vi "Autonomous Independent.vi"() -> ()   [LabVIEW 2015]
doc: "This VI is called when autonomous begins, and will automatically be terminated when autonomous ends. You can carry out timed or sensor driven robot movement independently without needing to return to the caller."
uses:
  Robot Global Data.vi
  <vilib>/Rock Robotics/Network Tables/NT Read Number.vi
  <vilib>/Rock Robotics/Network Tables/NT Read Boolean.vi
panel:
  out "Right Inches":dbl
  out "left inches":dbl
  out "Gyro Angle":dbl
  # "Be sure to right-click and choose Data Operations>>Make Current Value default if you want to save the array values with the VI"
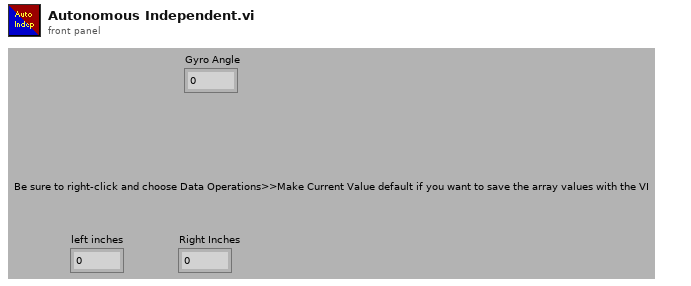
[diagram p1: front panel]
types:
  T1 = typedef "WPI_MotorControlDeviceRef.ctl" = cluster{"DeviceStatus":errorcluster, "Type":T2, "PWM":cluster{"PWM Channel":T3, "DeadBand":T4}, "CAN":cluster{"Device Number":u8, "Control Mode":T5, "Semaphore":T6, "Max Vout":dbl, "TalonSRX Control Mode":T7}, "Invert":bool}
  T2 = typedef "WPI_MotorControlType.ctl" = enum16{"PWM", "CAN", "CANTalonSRX"}
  T3 = typedef "FPGA_DIOPWMChannel.ctl" = enum8{"PWM 0", "PWM 1", "PWM 2", "PWM 3", "PWM 4", "PWM 5", "PWM 6", "PWM 7", "PWM 8", "PWM 9", "PWM MXP 0", "PWM MXP 1", "PWM MXP 2", "PWM MXP 3", "PWM MXP 4", "PWM MXP 5", "PWM MXP 6", "PWM MXP 7", "PWM MXP 8", "PWM MXP 9", "Invalid"}
  T4 = typedef "WPI_PWMDeadband.ctl" = cluster{"Name":string, "maxPositivePwm":i32, "minPositivePwm":i32, "centerPwm":i32, "maxNegativePwm":i32, "minNegativePwm":i32, "angularRange":u16}
  T5 = typedef "WPI_CANJaguar_ControlMode.ctl" = enum8{"Percent VBus", "Current", "Speed", "Position", "Voltage"}
  T6 = typedef "Semaphore RefNum" = refnum<k1>
  T7 = typedef "WPI_CANTalonSRX_APIControlMode.ctl" = enum8{"Percent VBus", "Speed", "Position", "Slave", "Unchanged / Invalid", "Voltage Compensation", "Current", "Motion Profile"}
  T8 = typedef "WPI_GyroDevRef.ctl" = cluster{"DevStatus":errorcluster, "Analog Channel":T9, "Offset":dbl, "Gain (VoltsPerDegree/Second)":dbl, "Gyro Type":enum16{"Analog", "XRS450"}, "Handle":i32, "SPI Bus":T10, "Device Found":bool, "Sample Rate":dbl, "Calibrate On Open":bool}
  T9 = typedef "FPGA_AIChannel.ctl" = enum8{"AI 0", "AI 1", "AI 2", "AI 3", "AI MXP 0", "AI MXP 1", "AI MXP 2", "AI MXP 3", "Invalid"}
  T10 = typedef "spi_bus.ctl" = enum16{"SPI On-Board, CS0", "SPI On-Board, CS1", "SPI On-Board, CS2", "SPI On-Board, CS3", "SPI MXP", "Invalid"}
  T11 = typedef "WPI_CANTalonSRX_GlobalStatus.ctl" = cluster{"Applied Throttle":dbl, "Module Enabled":bool, "CAN Error":errorcluster, "Closed Loop Error":dbl, "Forward Limit Switch Closed":bool, "Reverse Limit Switch Closed":bool, "Sensor Position":dbl, "Sensor Velocity":dbl, "Current":dbl, "Sticky Fault - Over Temp":bool, "Sticky Fault - Under Voltage":bool, "Sticky Fault - Forward Limit":bool, "Sticky Fault - Reverse Limit":bool, "Sticky Fault - Forward Soft Limit":bool, "Sticky Fault - Reverse Soft Limit":bool, "Brake is Enabled":bool, "Encoder Position":dbl, "Encoder Velocity":dbl, "Encoder Index Count":dbl, "Encoder A Pin State":bool, "Encoder B Pin State":bool, "Encoder Index Pin State":bool, "Analog In":dbl, "Analog In Velocity":dbl, "Temperature (C)":dbl, "Battery Voltage":dbl, "Control 5 Is Supported":bool, "Current Profile Slot Select":dbl, "Pos Div 8":bool, "Vel Div 4":bool, "Pulse Width Position":i32, "Pulse Width Velocity":i32, "Pulse Width Rise To Rise (us)":i32, "Pulse Width Rise To Fall (us)":i32, "Mot Prof Active Is Under Run":bool, "Mot Prof Active Has Under Run":bool, "Mot Prof Active Is Last":bool, "Mot Prof Active Velocity Only":bool, "Mot Prof Active Is Valid":bool, "Mot Prof Buffer Is Full":bool, "Mot Prof Active Profile Slot Select":i32, "Mot Prof NextID":i32, "Mot Prof Count":i32, "Mot Prof Active Velocity":dbl, "Mot Prof Active Position":dbl, "Mot Prof Output Enable":i32}
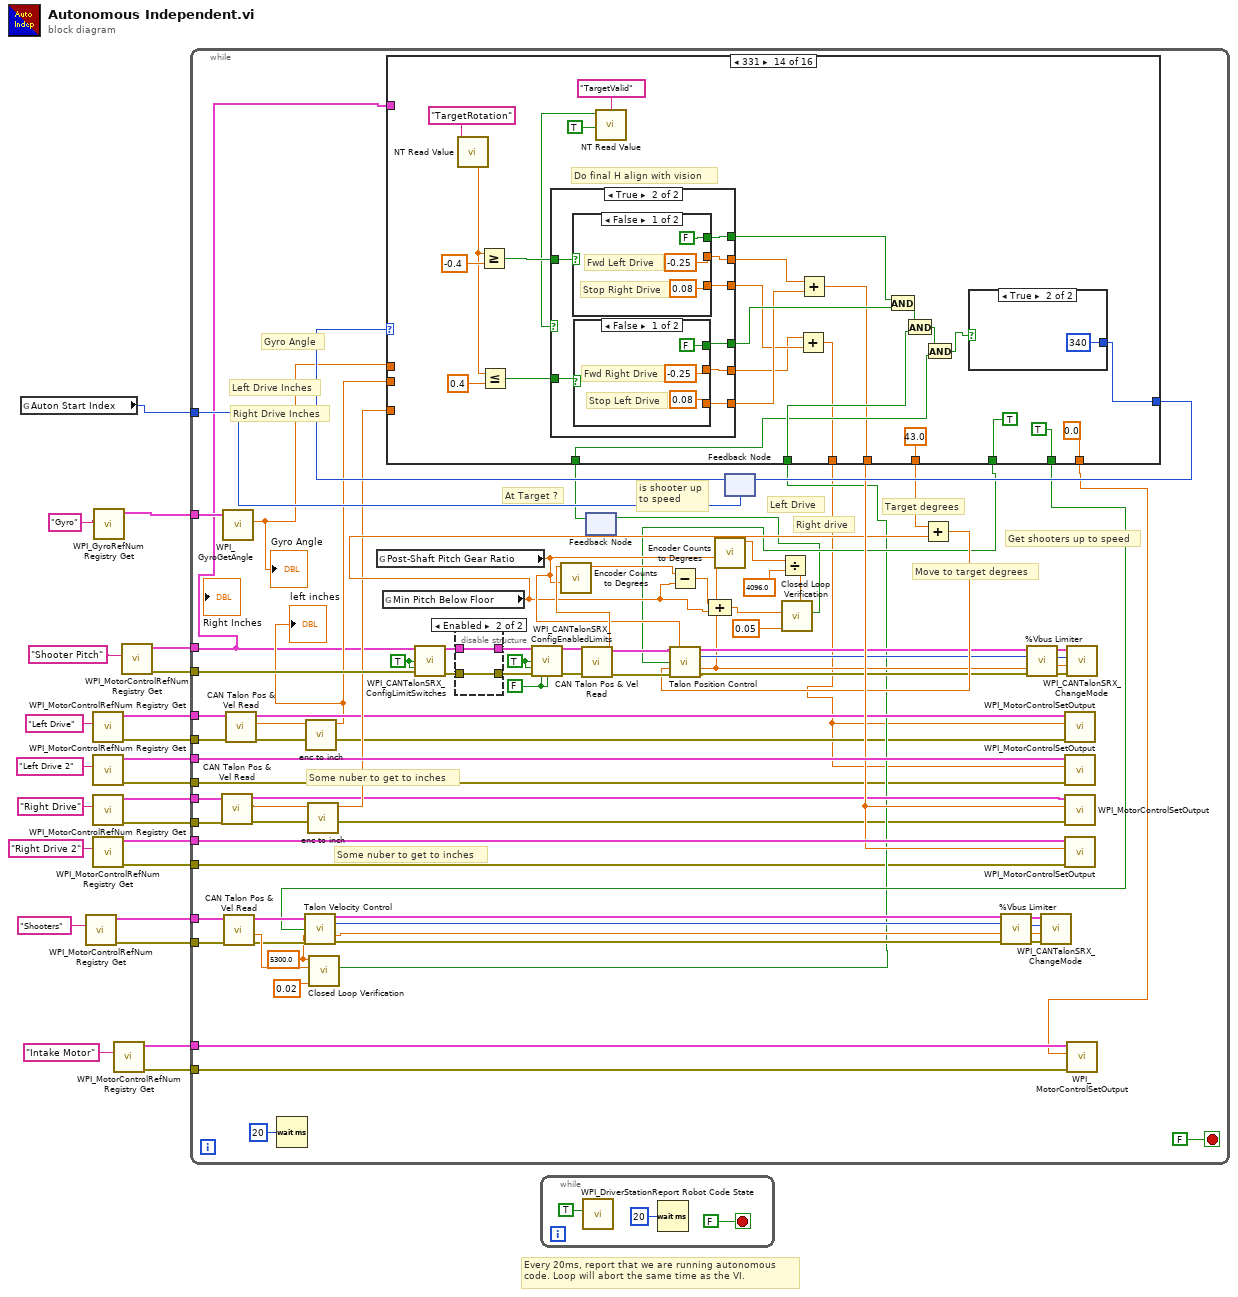
[diagram p0: block diagram]
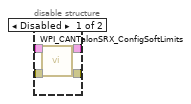
[diagram p2: hidden frame]
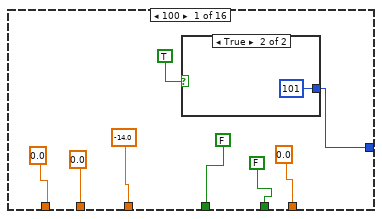
[diagram p3: hidden frame]
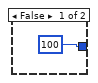
[diagram p4: hidden frame]
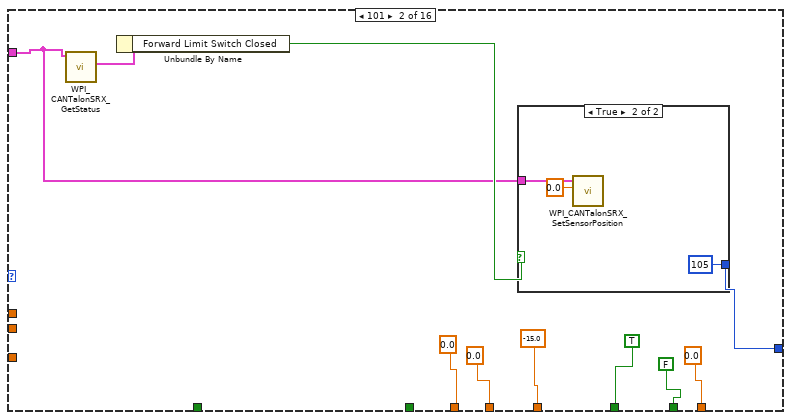
[diagram p5: hidden frame]
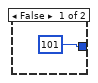
[diagram p6: hidden frame]
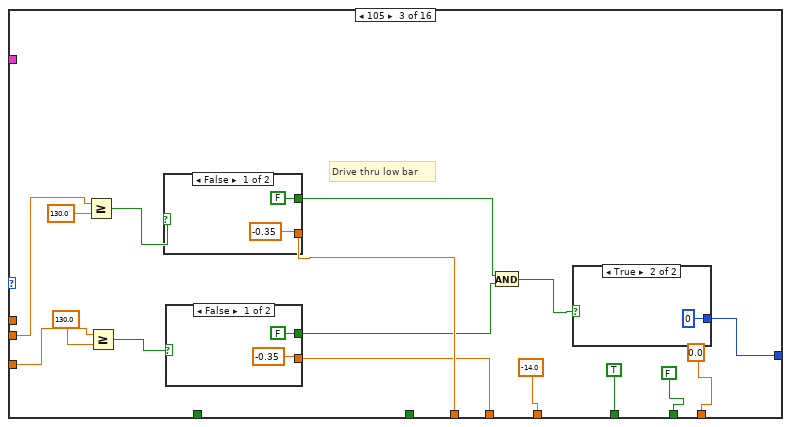
[diagram p7: hidden frame]
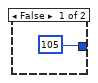
[diagram p8: hidden frame]
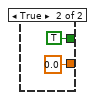
[diagram p9: hidden frame]
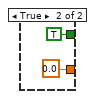
[diagram p10: hidden frame]
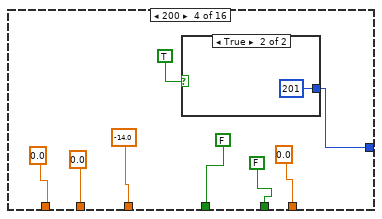
[diagram p11: hidden frame]
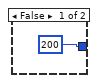
[diagram p12: hidden frame]
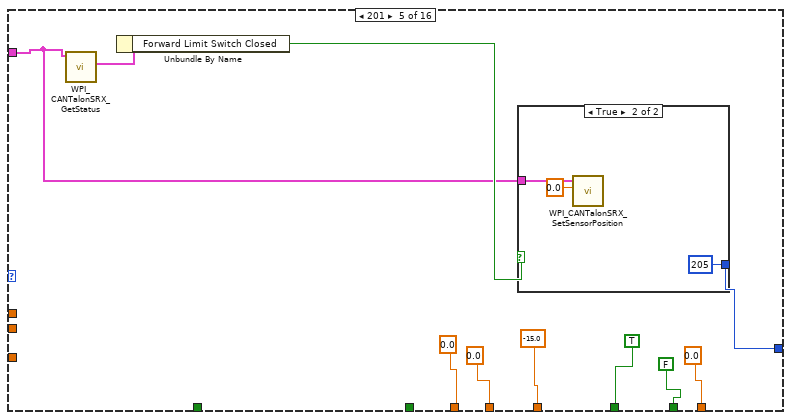
[diagram p13: hidden frame]
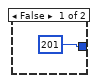
[diagram p14: hidden frame]
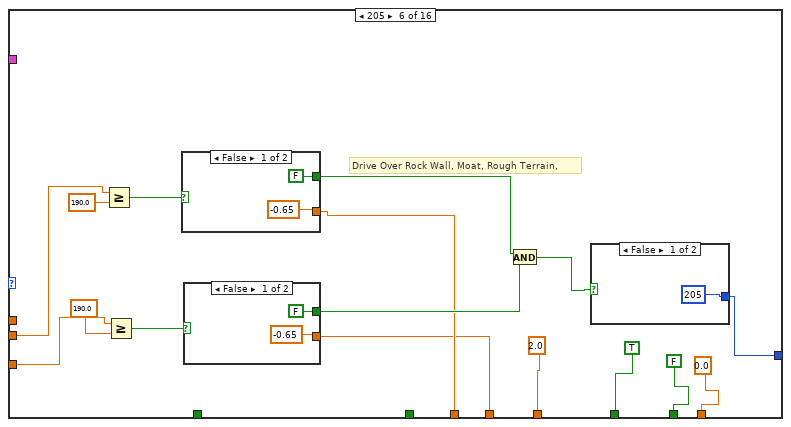
[diagram p15: hidden frame]
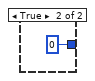
[diagram p16: hidden frame]
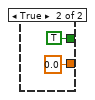
[diagram p17: hidden frame]
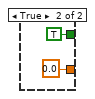
[diagram p18: hidden frame]
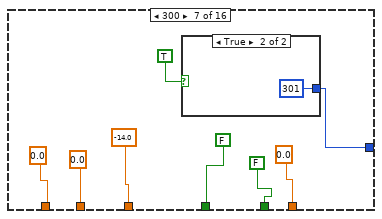
[diagram p19: hidden frame]
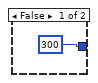
[diagram p20: hidden frame]
diagram:
  # "Every 20ms, report that we are running autonomous\ncode. Loop will abort the same time as the VI."
  n1 = global read "Robot Global Data.vi" "Auton Start Index"() -> (w1:i32)
  n2 = call <vilib>:"WPI_MotorControlRefNum Registry Get.vi"("refnum name"="Shooters") -> ("error out"=w7:errorcluster, "MotorControlDevRef"=w8:T1)  [unwired: 9 in]
  n3 = call <vilib>:"WPI_MotorControlRefNum Registry Get.vi"("refnum name"="Left Drive") -> ("error out"=w12:errorcluster, "MotorControlDevRef"=w13:T1)  [unwired: 9 in]
  n4 = call <vilib>:"WPI_MotorControlRefNum Registry Get.vi"("refnum name"="Left Drive 2") -> ("error out"=w2:errorcluster, "MotorControlDevRef"=w20:T1)  [unwired: 9 in]
  n5 = call <vilib>:"WPI_MotorControlRefNum Registry Get.vi"("refnum name"="Right Drive") -> ("error out"=w10:errorcluster, "MotorControlDevRef"=w11:T1)  [unwired: 9 in]
  n6 = call <vilib>:"WPI_MotorControlRefNum Registry Get.vi"("refnum name"="Right Drive 2") -> ("error out"=w3:errorcluster, "MotorControlDevRef"=w19:T1)  [unwired: 9 in]
  n7 = call <vilib>:"WPI_GyroRefNum Registry Get.vi"("refnum name"="Gyro") -> ("GyroDevRef"=w15:T8)  [unwired: 9 in, 1 out]
  n8 = call <vilib>:"WPI_MotorControlRefNum Registry Get.vi"("refnum name"="Intake Motor") -> ("error out"=w4:errorcluster, "MotorControlDevRef"=w5:T1)  [unwired: 9 in]
  n9 = call <vilib>:"WPI_MotorControlRefNum Registry Get.vi"("refnum name"="Shooter Pitch") -> ("error out"=w16:errorcluster, "MotorControlDevRef"=w17:T1)  [unwired: 9 in]
  n10 = while {
    tunnel: w1 -> [w101]
    tunnel: w15 -> [w100]
    tunnel: w13 -> [w58]
    tunnel: w20 -> [w98]
    tunnel: w11 -> [w55]
    tunnel: w19 -> [w97]
    tunnel: w17 -> [w26]
    tunnel: w16 -> [w88]
    tunnel: w12 -> [w59]
    tunnel: w10 -> [w53]
    tunnel: w8 -> [w50]
    tunnel: w7 -> [w49]
    tunnel: w5 -> [w33]
    tunnel: w4 -> [w32]
    tunnel: w3 -> [w31]
    tunnel: w2 -> [w29]
    stop <- FALSE stop-if-true
    w44 = 5300.0 ("Target")
    w89 = FALSE ("Forward Soft Limit Enable")
    w90 = TRUE ("Forward Limit Switch Enable")
    w95 = TRUE ("Forward Limit Switch Normally Open")
    # "is shooter up\nto speed"
    # "Get shooters up to speed"
    # "Right Drive Inches"
    # "Left Drive Inches"
    # "Gyro Angle"
    # "Some nuber to get to inches"
    # "Some nuber to get to inches"
    # "At Target ?"
    # "Move to target degrees"
    # "Target degrees"
    # "Right drive"
    # "Left Drive"
    n11 = call "CAN Talon Pos & Vel Read.vi"("error in (no error)"=w53, "CAN Talon SRX Ref"=w55) -> ("error out"=w30:errorcluster, "Sensor Position"=w52:dbl, "CAN Talon SRX Ref"=w54:T1)  [unwired: 5 in, 2 out]
    n12 = call <vilib>:"WPI_GyroGetAngle.vi"("GyroDevRef"=w100) -> ("Angle"=w99:dbl)  [unwired: 6 in, 4 out]
    "Gyro Angle" <- w99
    n13 = call "CAN Talon Pos & Vel Read.vi"("error in (no error)"=w49, "CAN Talon SRX Ref"=w50) -> ("error out"=w46:errorcluster, "Sensor Velocity"=w47:dbl, "CAN Talon SRX Ref"=w45:T1)  [unwired: 5 in, 2 out]
    n14 = call "CAN Talon Pos & Vel Read.vi"("error in (no error)"=w59, "CAN Talon SRX Ref"=w58) -> ("error out"=w28:errorcluster, "Sensor Position"=w57:dbl, "CAN Talon SRX Ref"=w56:T1)  [unwired: 5 in, 2 out]
    n15 = Wait (ms)(milliseconds to wait=u32 20) -> ()  [unwired: 1 out]
    n16 = call "enc to inch.vi"("Sensor position"=w57) -> ("Inches"=w51:dbl)  [unwired: 10 in]
    "left inches" <- w51
    n17 = call "enc to inch.vi"("Sensor position"=w52) -> ("Inches"=w60:dbl)  [unwired: 10 in]
    n18 = call "Closed Loop Verification.vi"("Allowable Error Factor"=0.02, "Actual"=w47, "Target"=w44) -> ("At Target w/in Allowable Error?"=w34:bool)  [unwired: 8 in]
    n19 = global read "Robot Global Data.vi" "Post-Shaft Pitch Gear Ratio"() -> (w78:dbl)
    n20 = global read "Robot Global Data.vi" "Min Pitch Below Floor"() -> (w75:dbl)
    n21 = call <vilib>:"WPI_CANTalonSRX_ConfigLimitSwitches.vi"("CAN Talon SRX Ref"=w26, "Forward Limit Switch Normally Open"=w95, "Reverse Limit Switch Normally Open"=w95, "error in (no error)"=w88) -> ("CAN Talon SRX Ref"=w94:T1, "error out"=w93:errorcluster)  [unwired: 10 in]
    n22 = disable-structure shown="Enabled" {
      disable-tunnel: w94 -> [w109 w111]
      disable-tunnel: w93 -> [w108 w110]
      disable-tunnel: [w107 w111] -> w92
      disable-tunnel: [w106 w110] -> w91
      frame Disabled {
        n23 = call <vilib>:"WPI_CANTalonSRX_ConfigSoftLimits.vi"("CAN Talon SRX Ref"=w109, "error in (no error)"=w108) -> ("CAN Talon SRX Ref"=w107:T1, "error out"=w106:errorcluster)  [unwired: 12 in]
      }
      frame Enabled {
      }
    }
    n24 = call <vilib>:"WPI_CANTalonSRX_ConfigEnabledLimits.vi"("CAN Talon SRX Ref"=w92, "Forward Limit Switch Enable"=w90, "Reverse Limit Switch Enable"=w90, "error in (no error)"=w91, "Forward Soft Limit Enable"=w89, "Reverse Soft Limit Enable"=w89) -> ("CAN Talon SRX Ref"=w87:T1, "error out"=w86:errorcluster)  [unwired: 8 in]
    n25 = call "CAN Talon Pos & Vel Read.vi"("error in (no error)"=w86, "CAN Talon SRX Ref"=w87) -> ("error out"=w82:errorcluster, "Sensor Position"=w85:dbl, "CAN Talon SRX Ref"=w83:T1)  [unwired: 5 in, 2 out]
    n26 = call "Encoder Counts to Degrees.vi"("Post-Shaft Gear Ratio"=w78, "Encoder Rotations"=w85) -> ("Degrees"=w84:dbl)  [unwired: 9 in]
    n27 = feedback #1() -> (w69:bool)  [unwired: 1 in]
    n28 = Subtract(x=w84, y=w75) -> (x-y=w81:dbl)
    n29 = Compound Arithmetic op=ADD(w81, w75) -> (w80:dbl)
    n30 = feedback #2(w101) -> (w102:i64)
    n31 = case shown="331" w102 {
      tunnel: [w117 w129 w139 w167 w179 w188 w217 w229 w238 w264 w291 w317 w345 w392 w438 i64 0 ("milliseconds to wait")] -> w103
      tunnel: w99 -> [_ _ _ _ _ _ _ _ _ _ _ _ _ _ _ _]
      tunnel: [0.0 ("Angle") 0.0 ("Angle") w146 0.0 ("Angle") 0.0 ("Angle") w192 0.0 ("Angle") 0.0 ("Angle") w242 w268 w295 w321 w349 w369 w442 0.0 ("Angle")] -> w25
      tunnel: [0.0 ("Angle") 0.0 ("Angle") w145 0.0 ("Angle") 0.0 ("Angle") w191 0.0 ("Angle") 0.0 ("Angle") w241 w267 w294 w320 w348 w368 w441 0.0 ("Angle")] -> w96
      tunnel: [-14.0 ("Angle") -15.0 ("Angle") -14.0 ("Angle") -14.0 ("Angle") -15.0 ("Angle") 2.0 ("Angle") -14.0 ("Angle") -15.0 ("Angle") -14.0 ("Angle") 43.0 ("Angle") 43.0 ("Angle") 43.0 ("Angle") 43.0 ("Angle") 43.0 ("Angle") 43.0 ("Angle") -15.8 ("Angle")] -> w76
      tunnel: [FALSE ("Forward Soft Limit Enable") TRUE ("Forward Soft Limit Enable") TRUE ("Forward Soft Limit Enable") FALSE ("Forward Soft Limit Enable") TRUE ("Forward Soft Limit Enable") TRUE ("Forward Soft Limit Enable") FALSE ("Forward Soft Limit Enable") TRUE ("Forward Soft Limit Enable") TRUE ("Forward Soft Limit Enable") TRUE ("Forward Soft Limit Enable") TRUE ("Forward Soft Limit Enable") TRUE ("Forward Soft Limit Enable") TRUE ("Forward Soft Limit Enable") TRUE ("Forward Soft Limit Enable") TRUE ("Forward Soft Limit Enable") FALSE ("Forward Soft Limit Enable")] -> w74
      tunnel: w69 -> [_ _ _ _ _ _ _ _ _ _ _ w316 w341 w385 w431 _]
      tunnel: w51 -> [_ _ w147 _ _ w193 _ _ w243 w269 w296 w322 w350 _ w443 _]
      tunnel: w60 -> [_ _ w148 _ _ w194 _ _ w244 w270 w297 w323 w351 _ w444 _]
      tunnel: [FALSE FALSE FALSE FALSE FALSE FALSE FALSE FALSE FALSE FALSE FALSE ("Forward Soft Limit Enable") FALSE ("Forward Soft Limit Enable") TRUE ("Forward Soft Limit Enable") TRUE ("Forward Soft Limit Enable") TRUE ("Forward Soft Limit Enable") FALSE ("Forward Soft Limit Enable")] -> w43
      tunnel: w34 -> [_ _ _ _ _ _ _ _ _ _ _ _ _ w390 w436 _]
      tunnel: [0.0 ("Angle") 0.0 ("Angle") 0.0 ("Angle") 0.0 ("Angle") 0.0 ("Angle") 0.0 ("Angle") 0.0 ("Angle") 0.0 ("Angle") 0.0 ("Angle") 0.0 ("Angle") 0.0 ("Angle") 0.0 ("Angle") 0.0 ("Angle") 0.0 ("Angle") 1.0 ("Angle") 0.0 ("Angle")] -> w27
      tunnel: w26 -> [_ w122 _ _ w172 _ _ w222 _ _ _ _ _ _ _ _]
      frame 100 {
        n32 = case shown="True" TRUE {
          tunnel: [i64 100 ("milliseconds to wait") i64 101 ("milliseconds to wait")] -> w117
          frame False {
          }
          frame True {
          }
        }
      }
      frame 101 {
        n33 = call <vilib>:"WPI_CANTalonSRX_GetStatus.vi"("CAN Talon SRX Ref"=w122) -> ("Talon SRX Status"=w124:T11)  [unwired: 8 in, 2 out]
        n34 = Unbundle By Name(w124) -> ("Forward Limit Switch Closed"=w123:bool)
        n35 = case shown="True" w123 {
          tunnel: [i64 101 ("milliseconds to wait") i64 105 ("milliseconds to wait")] -> w129
          tunnel: w122 -> [_ w134]
          frame False {
          }
          frame True {
            n36 = call <vilib>:"WPI_CANTalonSRX_SetSensorPosition.vi"("New Sensor Position"=0.0, "CAN Talon SRX Ref"=w134) -> ()  [unwired: 8 in, 2 out]
          }
        }
      }
      frame 105 {
        # "Drive thru low bar"
        n37 = Greater Or Equal?(x=w147, y=130.0) -> (x >= y?=w151:bool)
        n38 = Greater Or Equal?(x=w148, y=130.0) -> (x >= y?=w150:bool)
        n39 = case shown="False" w151 {
          tunnel: [-0.35 ("y") 0.0 ("y")] -> w146
          tunnel: [FALSE TRUE] -> w142
          frame False {
          }
          frame True {
          }
        }
        n40 = case shown="False" w150 {
          tunnel: [-0.35 ("y") 0.0 ("y")] -> w145
          tunnel: [FALSE TRUE] -> w141
          frame False {
          }
          frame True {
          }
        }
        n41 = And(x=w142, y=w141) -> (x .and. y?=w140:bool)
        n42 = case shown="True" w140 {
          tunnel: [i64 105 ("milliseconds to wait") i64 0 ("milliseconds to wait")] -> w139
          frame False {
          }
          frame True {
          }
        }
      }
      frame 200 {
        n43 = case shown="True" TRUE {
          tunnel: [i64 200 ("milliseconds to wait") i64 201 ("milliseconds to wait")] -> w167
          frame False {
          }
          frame True {
          }
        }
      }
      frame 201 {
        n44 = call <vilib>:"WPI_CANTalonSRX_GetStatus.vi"("CAN Talon SRX Ref"=w172) -> ("Talon SRX Status"=w174:T11)  [unwired: 8 in, 2 out]
        n45 = Unbundle By Name(w174) -> ("Forward Limit Switch Closed"=w173:bool)
        n46 = case shown="True" w173 {
          tunnel: [i64 201 ("milliseconds to wait") i64 205 ("milliseconds to wait")] -> w179
          tunnel: w172 -> [_ w184]
          frame False {
          }
          frame True {
            n47 = call <vilib>:"WPI_CANTalonSRX_SetSensorPosition.vi"("New Sensor Position"=0.0, "CAN Talon SRX Ref"=w184) -> ()  [unwired: 8 in, 2 out]
          }
        }
      }
      frame 205 {
        # "Drive Over Rock Wall, Moat, Rough Terrain,"
        n48 = Greater Or Equal?(x=w193, y=190.0) -> (x >= y?=w200:bool)
        n49 = Greater Or Equal?(x=w194, y=190.0) -> (x >= y?=w199:bool)
        n50 = case shown="False" w200 {
          tunnel: [-0.65 ("y") 0.0 ("y")] -> w192
          tunnel: [FALSE TRUE] -> w197
          frame False {
          }
          frame True {
          }
        }
        n51 = case shown="False" w199 {
          tunnel: [-0.65 ("y") 0.0 ("y")] -> w191
          tunnel: [FALSE TRUE] -> w196
          frame False {
          }
          frame True {
          }
        }
        n52 = And(x=w197, y=w196) -> (x .and. y?=w195:bool)
        n53 = case shown="False" w195 {
          tunnel: [i64 205 ("milliseconds to wait") i64 0 ("milliseconds to wait")] -> w188
          frame False {
          }
          frame True {
          }
        }
      }
      frame 300 {
        n54 = case shown="True" TRUE {
          tunnel: [i64 300 ("milliseconds to wait") i64 301 ("milliseconds to wait")] -> w217
          frame False {
          }
          frame True {
          }
        }
      }
      frame 301 {
        n55 = call <vilib>:"WPI_CANTalonSRX_GetStatus.vi"("CAN Talon SRX Ref"=w222) -> ("Talon SRX Status"=w224:T11)  [unwired: 8 in, 2 out]
        n56 = Unbundle By Name(w224) -> ("Forward Limit Switch Closed"=w223:bool)
        n57 = case shown="True" w223 {
          tunnel: [i64 301 ("milliseconds to wait") i64 305 ("milliseconds to wait")] -> w229
          tunnel: w222 -> [_ w234]
          frame False {
          }
          frame True {
            n58 = call <vilib>:"WPI_CANTalonSRX_SetSensorPosition.vi"("New Sensor Position"=0.0, "CAN Talon SRX Ref"=w234) -> ()  [unwired: 8 in, 2 out]
          }
        }
      }
      frame 305 {
        # "Driver Thru Low bar Then..."
        n59 = Greater Or Equal?(x=w243, y=110.0) -> (x >= y?=w250:bool)
        n60 = Greater Or Equal?(x=w244, y=110.0) -> (x >= y?=w249:bool)
        n61 = case shown="False" w250 {
          tunnel: [-0.35 ("y") 0.0 ("y")] -> w242
          tunnel: [FALSE TRUE] -> w247
          frame False {
          }
          frame True {
          }
        }
        n62 = case shown="False" w249 {
          tunnel: [-0.35 ("y") 0.0 ("y")] -> w241
          tunnel: [FALSE TRUE] -> w246
          frame False {
          }
          frame True {
          }
        }
        n63 = And(x=w247, y=w246) -> (x .and. y?=w245:bool)
        n64 = case shown="True" w245 {
          tunnel: [i64 305 ("milliseconds to wait") i64 310 ("milliseconds to wait")] -> w238
          frame False {
          }
          frame True {
          }
        }
      }
      frame 310 {
        # "Then turn towards Tower Then..."
        n65 = Greater Or Equal?(x=w269, y=194.0) -> (x >= y?=w276:bool)
        n66 = Greater Or Equal?(x=w270, y=110.0) -> (x >= y?=w275:bool)
        n67 = case shown="False" w276 {
          tunnel: [-0.5 ("y") 0.0 ("y")] -> w268
          tunnel: [FALSE TRUE] -> w273
          frame False {
          }
          frame True {
          }
        }
        n68 = case shown="False" w275 {
          tunnel: [-0.5 ("y") 0.0 ("y")] -> w267
          tunnel: [FALSE TRUE] -> w272
          frame False {
          }
          frame True {
          }
        }
        n69 = And(x=w273, y=w272) -> (x .and. y?=w271:bool)
        n70 = case shown="True" w271 {
          tunnel: [i64 310 ("milliseconds to wait") i64 320 ("milliseconds to wait")] -> w264
          frame False {
          }
          frame True {
          }
        }
      }
      frame 320 {
        # "Then set shooter down"
        n71 = Greater Or Equal?(x=w296, y=194.0) -> (x >= y?=w300:bool)
        n72 = Greater Or Equal?(x=w297, y=110.0) -> (x >= y?=w299:bool)
        n73 = case shown="False" w300 {
          tunnel: [-0.35 ("y") 0.0 ("y")] -> w295
          tunnel: [FALSE TRUE] -> _
          frame False {
          }
          frame True {
          }
        }
        n74 = case shown="False" w299 {
          tunnel: [-0.35 ("y") 0.0 ("y")] -> w294
          tunnel: [FALSE TRUE] -> _
          frame False {
          }
          frame True {
          }
        }
        n75 = case shown="True" TRUE {
          tunnel: [i64 320 ("milliseconds to wait") i64 325 ("milliseconds to wait")] -> w291
          frame False {
          }
          frame True {
          }
        }
      }
      frame 325 {
        # "Then lift shooter up"
        n76 = Greater Or Equal?(x=w322, y=194.0) -> (x >= y?=w328:bool)
        n77 = Greater Or Equal?(x=w323, y=110.0) -> (x >= y?=w327:bool)
        n78 = case shown="False" w328 {
          tunnel: [-0.35 ("y") 0.0 ("y")] -> w321
          tunnel: [FALSE TRUE] -> w325
          frame False {
          }
          frame True {
          }
        }
        n79 = case shown="False" w327 {
          tunnel: [-0.35 ("y") 0.0 ("y")] -> w320
          tunnel: [FALSE TRUE] -> w324
          frame False {
          }
          frame True {
          }
        }
        n80 = And(x=w325, y=w324) -> (x .and. y?=w315:bool)
        n81 = And(x=w315, y=w316) -> (x .and. y?=w314:bool)
        n82 = case shown="True" w314 {
          tunnel: [i64 325 ("milliseconds to wait") i64 330 ("milliseconds to wait")] -> w317
          frame False {
          }
          frame True {
          }
        }
      }
      frame 330 {
        # "Then lift shooter up and get moters going"
        n83 = Greater Or Equal?(x=w350, y=194.0) -> (x >= y?=w356:bool)
        n84 = Greater Or Equal?(x=w351, y=110.0) -> (x >= y?=w355:bool)
        n85 = case shown="False" w356 {
          tunnel: [-0.5 ("y") 0.0 ("y")] -> w349
          tunnel: [FALSE TRUE] -> w353
          frame False {
          }
          frame True {
          }
        }
        n86 = case shown="False" w355 {
          tunnel: [-0.5 ("y") 0.0 ("y")] -> w348
          tunnel: [FALSE TRUE] -> w352
          frame False {
          }
          frame True {
          }
        }
        n87 = And(x=w353, y=w352) -> (x .and. y?=w340:bool)
        n88 = And(x=w340, y=w341) -> (x .and. y?=w342:bool)
        n89 = case shown="True" w342 {
          tunnel: [i64 330 ("milliseconds to wait") i64 331 ("milliseconds to wait")] -> w345
          frame False {
          }
          frame True {
          }
        }
      }
      frame 331 {
        # "Do final H align with vision"
        n90 = call-poly <vilib>:"NT Read Value.vi"("Name"="TargetRotation") -> ("Numeric"=w381:dbl)  [unwired: 9 in, 1 out]
        n91 = Greater Or Equal?(x=w381, y=-0.4) -> (x >= y?=w377:bool)
        n92 = Less Or Equal?(x=w381, y=0.4) -> (x <= y?=w376:bool)
        n93 = call-poly <vilib>:"NT Read Value.vi"("Default Value"=TRUE, "Name"="TargetValid") -> ("Boolean"=w375:bool)  [unwired: 8 in, 1 out]
        n94 = case shown="True" w375 {
          tunnel: [TRUE w408] -> w378
          tunnel: w377 -> [_ w407]
          tunnel: w376 -> [_ w406]
          tunnel: [TRUE w405] -> w374
          tunnel: [0.0 ("y") w404] -> w371
          tunnel: [0.0 ("y") w403] -> w370
          tunnel: [0.0 ("y") w402] -> w372
          tunnel: [0.0 ("y") w401] -> w373
          frame False {
          }
          frame True {
            n95 = case shown="False" w407 {
              tunnel: [-0.25 ("y") 0.0 ("y")] -> w403
              tunnel: [FALSE TRUE] -> w408
              tunnel: [0.08 ("y") 0.0 ("y")] -> w402
              frame False {
                # "Fwd Left Drive"
                # "Stop Right Drive"
              }
              frame True {
              }
            }
            n96 = case shown="False" w406 {
              tunnel: [-0.25 ("y") 0.0 ("y")] -> w404
              tunnel: [FALSE TRUE] -> w405
              tunnel: [0.08 ("y") 0.0 ("y")] -> w401
              frame False {
                # "Fwd Right Drive"
                # "Stop Left Drive"
              }
              frame True {
              }
            }
          }
        }
        n97 = Add(x=w371, y=w372) -> (x+y=w369:dbl)
        n98 = Add(x=w370, y=w373) -> (x+y=w368:dbl)
        n99 = And(x=w378, y=w374) -> (x .and. y?=w389:bool)
        n100 = And(x=w389, y=w390) -> (x .and. y?=w387:bool)
        n101 = And(x=w387, y=w385) -> (x .and. y?=w386:bool)
        n102 = case shown="True" w386 {
          tunnel: [i64 331 ("milliseconds to wait") i64 340 ("milliseconds to wait")] -> w392
          frame False {
          }
          frame True {
          }
        }
      }
      frame 340 {
        # "Shoot!"
        n103 = Greater Or Equal?(x=w443, y=194.0) -> (x >= y?=w449:bool)
        n104 = Greater Or Equal?(x=w444, y=110.0) -> (x >= y?=w448:bool)
        n105 = case shown="False" w449 {
          tunnel: [-0.35 ("y") 0.0 ("y")] -> w442
          tunnel: [FALSE TRUE] -> w446
          frame False {
          }
          frame True {
          }
        }
        n106 = case shown="False" w448 {
          tunnel: [-0.35 ("y") 0.0 ("y")] -> w441
          tunnel: [FALSE TRUE] -> w445
          frame False {
          }
          frame True {
          }
        }
        n107 = Tick Count (ms)() -> (millisecond timer value=w425:u32)
        n108 = First Call?() -> (First Call?: T/F=w429:bool)
        n109 = feedback #3() -> (w428:u32)  [unwired: 1 in]
        n110 = case shown="False" w429 {
          tunnel: w425 -> [_ w452]
          tunnel: [w451 w452] -> w426
          tunnel: w428 -> [w451 _]
          frame False {
          }
          frame True {
          }
        }
        n111 = feedback-in #3(w426) -> ()
        n112 = Subtract(x=w425, y=w426) -> (x-y=w427:u32)
        n113 = Greater?(x=w427, y=u32 1000) -> (0:w423:bool)
        n114 = And(x=w446, y=w445) -> (x .and. y?=w435:bool)
        n115 = And(x=w435, y=w436) -> (x .and. y?=w433:bool)
        n116 = And(x=w433, y=w431) -> (x .and. y?=w432:bool)
        n117 = And(x=w423, y=w432) -> (x .and. y?=w430:bool)
        n118 = case shown="True" w430 {
          tunnel: [i64 340 ("milliseconds to wait") i64 0 ("milliseconds to wait")] -> w438
          frame False {
          }
          frame True {
          }
        }
      }
      frame 0, Default {
      }
    }
    n119 = call "Talon Velocity Control.vi"("CAN Talon SRX Ref"=w45, "Run to Speed?"=w43, "TargetSpeedRPM"=w44, "error in (no error)"=w46) -> ("CAN Talon SRX Ref"=w38:T1, "Control Mode"=w36:T7, "Motor Set"=w35:dbl, "error out"=w37:errorcluster)  [unwired: 8 in]
    n120 = feedback-in #2(w103) -> ()
    n121 = Add(x=w76, y=w75) -> (x+y=w77:dbl)
    n122 = call "Talon Position Control.vi"("CAN Talon SRX Ref"=w83, "Post-Shaft Gear Ratio"=w78, "Move to Target?"=w74, "Target Degrees"=w77, "error in (no error)"=w82) -> ("CAN Talon SRX Ref"=w64:T1, "Control Mode"=w63:T7, "Encoder Count Target"=w62:dbl, "error out"=w61:errorcluster)  [unwired: 7 in]
    n123 = call "Encoder Counts to Degrees.vi"("Post-Shaft Gear Ratio"=w78, "Encoder Rotations"=w62) -> ("Degrees"=w72:dbl)  [unwired: 9 in]
    n124 = Divide(x=w72, y=4096.0) -> (x/y=w71:dbl)
    n125 = call "Closed Loop Verification.vi"("Allowable Error Factor"=0.05, "Actual"=w80, "Target"=w71) -> ("At Target w/in Allowable Error?"=w70:bool)  [unwired: 8 in]
    n126 = feedback-in #1(w70) -> ()
    n127 = call "%Vbus Limiter.vi"("error in (no error)"=w37, "Motor Set In"=w35, "Control Mode"=w36, "CAN Talon SRX Ref"=w38) -> ("error out"=w39:errorcluster, "Motor Set Out"=w40:dbl, "Control Mode"=w41:T7, "CAN Talon SRX Ref"=w42:T1)  [unwired: 4 in]
    n128 = call "%Vbus Limiter.vi"("error in (no error)"=w61, "Motor Set In"=w62, "Control Mode"=w63, "CAN Talon SRX Ref"=w64) -> ("error out"=w68:errorcluster, "Motor Set Out"=w67:dbl, "Control Mode"=w66:T7, "CAN Talon SRX Ref"=w65:T1)  [unwired: 4 in]
    n129 = call <vilib>:"WPI_CANTalonSRX_ChangeMode.vi"("error in (no error)"=w39, "Output"=w40, "Control Mode"=w41, "CAN Talon SRX Ref"=w42) -> ()  [unwired: 6 in, 2 out]
    n130 = call <vilib>:"WPI_MotorControlSetOutput.vi"("error in (no error)"=w28, "Output"=w25, "MotorControlDevRef"=w56) -> ()  [unwired: 6 in, 3 out]
    n131 = call <vilib>:"WPI_MotorControlSetOutput.vi"("error in (no error)"=w29, "Output"=w25, "MotorControlDevRef"=w98) -> ()  [unwired: 6 in, 3 out]
    n132 = call <vilib>:"WPI_MotorControlSetOutput.vi"("error in (no error)"=w30, "Output"=w96, "MotorControlDevRef"=w54) -> ()  [unwired: 6 in, 3 out]
    n133 = call <vilib>:"WPI_MotorControlSetOutput.vi"("error in (no error)"=w31, "Output"=w96, "MotorControlDevRef"=w97) -> ()  [unwired: 6 in, 3 out]
    n134 = call <vilib>:"WPI_CANTalonSRX_ChangeMode.vi"("error in (no error)"=w68, "Output"=w67, "Control Mode"=w66, "CAN Talon SRX Ref"=w65) -> ()  [unwired: 6 in, 2 out]
    n135 = call <vilib>:"WPI_MotorControlSetOutput.vi"("error in (no error)"=w32, "Output"=w27, "MotorControlDevRef"=w33) -> ()  [unwired: 6 in, 3 out]
  }
  n136 = while {
    stop <- FALSE stop-if-true
    n137 = call <vilib>:"WPI_DriverStationReport Robot Code State.vi"("Autonomous"=TRUE) -> ()  [unwired: 10 in, 1 out]
    n138 = Wait (ms)(milliseconds to wait=u32 20) -> ()  [unwired: 1 out]
  }
